vi "sv_UFF58 Read Data Format.vi"(0 "function refnum":refnum<k20>, 11 "error in (no error)":errorcluster) -> (3 "data form":T1={"ordinate data type"=4, "number of data values/pairs"=0, "abscissa spacing"=enum."uneven", "abscissa minimum"=0.0, "abscissa increment"=0.0} {"ordinate data type" items=["real single precision"=2, "real double precision"=4, "complex single precision"=5, "complex double precision"=6]}, 4 "dup function refnum":refnum<k20>, 6 "even":bool=TRUE, 10 "real":bool=TRUE, 15 "error out":errorcluster)   [LabVIEW 2017, in "SoundVib_UFF58.lvlib"]
doc: "This VI extracts the values of <B>OrdinateDatatype</B> and <B>AbscissaSpacing</B> from the X channel to check the function data type (real, complex) and data spacing (even, uneven). If <B>real</B> is false, it implies the data is complex. If <B>even</B> is false, it implies the data is uneven. It also returns an error if the data doesn't match the uff standard."
uses:
  <vilib>/addons/Sound and Vibration/svt_UFF58/SoundVib_UFF58.lvlib
  <vilib>/addons/Sound and Vibration/svt_UFF58/subVIs/sv_UFF58 Data Form.ctl
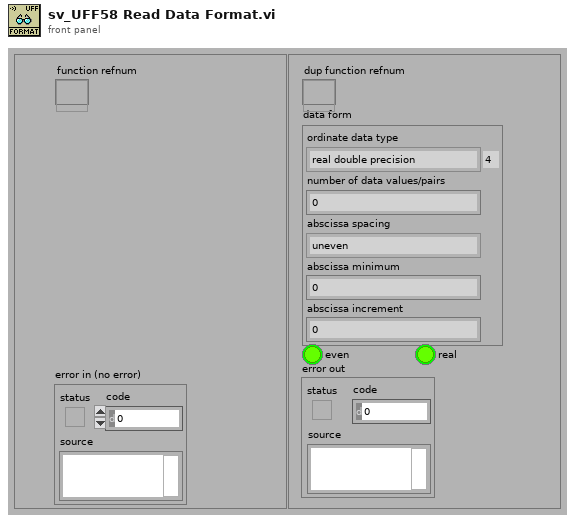
[diagram p1: front panel]
types:
  T1 = typedef "SoundVib_UFF58.lvlib/sv_UFF58 Data Form.ctl" = cluster{"ordinate data type":u16, "number of data values/pairs":i32, "abscissa spacing":enum16{"uneven", "even"}, "abscissa minimum":dbl, "abscissa increment":dbl}
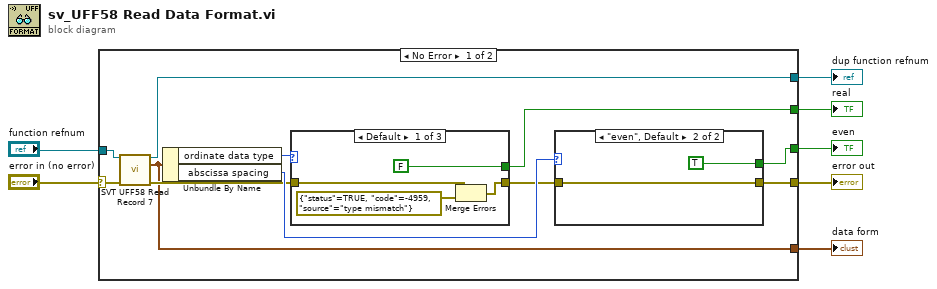
[diagram p0: block diagram]
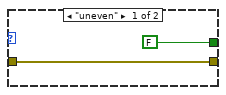
[diagram p2: hidden frame]
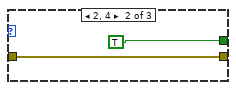
[diagram p3: hidden frame]
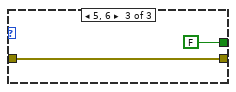
[diagram p4: hidden frame]
diagram:
  n1 = case shown="No Error" "error in (no error)" {
    selector: "error in (no error)" -> [w17 w31]
    tunnel: [w14 _] -> w7
    tunnel: [w10 _] -> w6
    tunnel: [w16 w32] -> w1
    tunnel: [w11 w31] -> w5
    tunnel: "function refnum" -> [w18 w32]
    tunnel: [w9 _] -> w3
    frame No Error {
      n2 = call <vilib>:"SVT UFF58 Read Record 7.vi"("function refnum"=w18, "error in (no error)"=w17) -> ("dup function refnum"=w16:refnum<k20>, "data form"=w9:T1, "error out"=w12:errorcluster)  [unwired: 11 in]
      n3 = Unbundle By Name(w9) -> ("ordinate data type"=w15:u16, "abscissa spacing"=w13:enum16{"uneven", "even"})
      n4 = case shown="Default" w15 {
        tunnel: [FALSE TRUE FALSE] -> w14
        tunnel: w12 -> [w25 w27 w29]
        tunnel: [w23 w27 w29] -> w8
        frame Default {
          n5 = Merge Errors(w25, errorcluster {"status"=TRUE, "code"=-4959, "source"="type mismatch"} ("error in 2 (no error)")) -> (w23:errorcluster)
        }
        frame 2, 4 {
        }
        frame 5, 6 {
        }
      }
      n6 = case shown="\"even\", Default" w13 {
        tunnel: w8 -> [w19 w21]
        tunnel: [w19 w21] -> w11
        tunnel: [FALSE TRUE] -> w10
        frame "uneven" {
        }
        frame "even", Default {
        }
      }
    }
    frame Error {
    }
  }
  "even" <- w6
  "real" <- w7
  "error out" <- w5
  "data form" <- w3
  "dup function refnum" <- w1
